vi "Read Type Name Handling.vi"(8 "error in (no error)":errorcluster, 11 "Flatten To JSON Object in":refnum<class "Flatten To JSON Object.lvclass">) -> (0 "error out":errorcluster, 2 "Type Name Handling":T1, 3 "Flatten To JSON Object out":refnum<class "Flatten To JSON Object.lvclass">)   [LabVIEW 2017, in "Flatten To JSON Object.lvclass"]
uses:
  Flatten To JSON Object.lvclass
  Type Name Handling.ctl
  Flatten To JSON Object.lvclass/Flatten To JSON Object.ctl
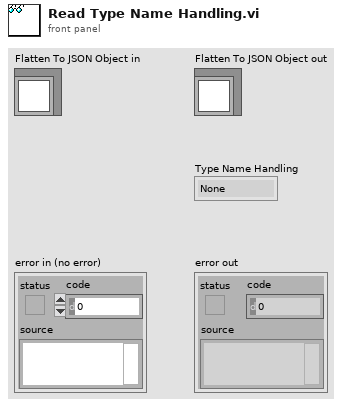
[diagram p1: front panel]
types:
  T1 = typedef "Flatten To JSON Object.lvclass/Type Name Handling.ctl" = enum16{"None", "Inline", "Separate"}
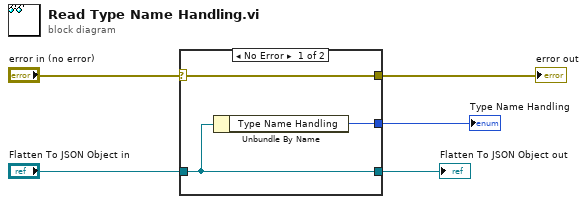
[diagram p0: block diagram]
diagram:
  n1 = case shown="No Error" "error in (no error)" {
    selector: "error in (no error)" -> [w8 w9]
    tunnel: [w8 w9] -> w4
    tunnel: [w7 w10] -> w2
    tunnel: "Flatten To JSON Object in" -> [w7 w10]
    tunnel: [w6 _] -> w1
    frame No Error {
      n2 = Unbundle By Name(w7) -> ("Type Name Handling"=w6:T1)
    }
    frame Error {
    }
  }
  "error out" <- w4
  "Flatten To JSON Object out" <- w2
  "Type Name Handling" <- w1
